vi "Hermite Interpolation 1D.vi"(9 "xi":dbl[](array[numeric]) format="%_6g", 10 "X":dbl[](array[numeric]), 11 "Y":dbl[](array[numeric])) -> (0 "error":i32, 1 "piecewise polynomial":T1 {"x locations" format="%.4g"; "coefficients" format="%.4g"}, 3 "yi":dbl[](array[numeric]) format="%_6g")   [LabVIEW 2010, in "NI_Gmath.lvlib"]
doc: "Performs one-dimensional interpolation using the cubic Hermite interpolation method based on the lookup table defined by <B>X</B> and <B>Y</B>."
uses:
  NI_Gmath.lvlib
  in_piecewise interp poly control.ctl
panel:
  # "Hermite Interpolation 1D"
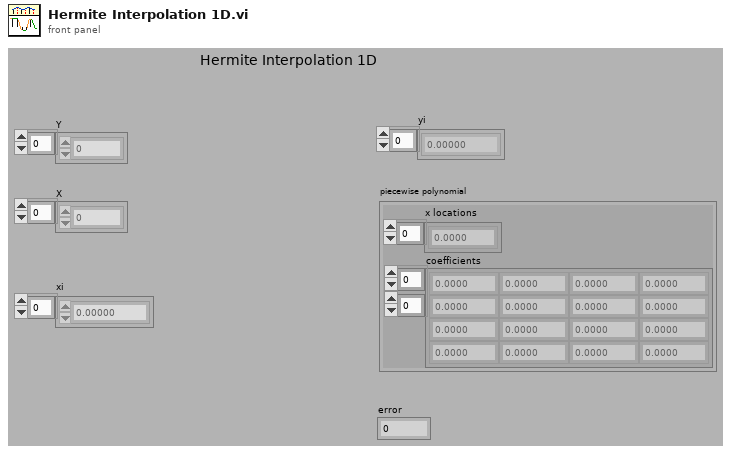
[diagram p1: front panel]
types:
  T1 = typedef "NI_Gmath.lvlib/in_piecewise interp poly control.ctl" = cluster{"x locations":dbl[], "coefficients":dbl[][]}
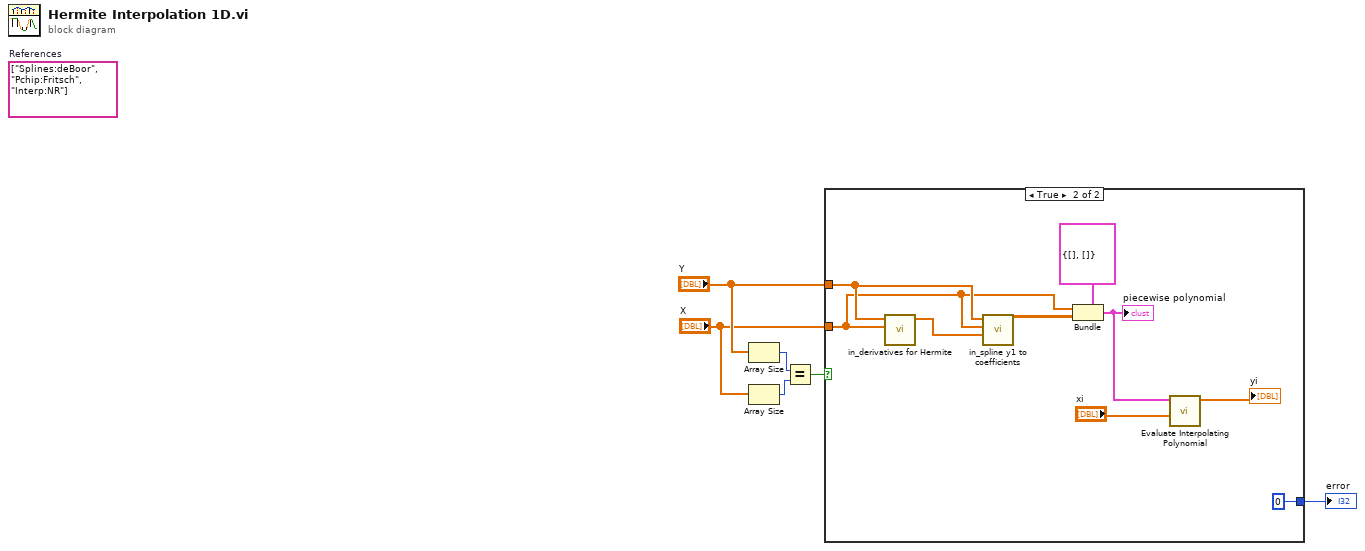
[diagram p0: block diagram]
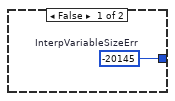
[diagram p2: hidden frame]
diagram:
  (unwired) string[] ["Splines:deBoor", "Pchip:Fritsch", "Interp:NR"]  # References
  n1 = Array Size(array="Y") -> (size(s)=w6:i32)
  n2 = Array Size(array="X") -> (size(s)=w5:i32)
  n3 = Equal?(x=w6, y=w5) -> (x = y?=w2:bool)
  n4 = case shown="True" w2 {
    tunnel: "Y" -> [_ w10]
    tunnel: "X" -> [_ w9]
    tunnel: [w7 0 ("error")] -> w1
    frame False {
      w7 = -20145  # InterpVariableSizeErr
    }
    frame True {
      n5 = call "in_derivatives for Hermite.vi"("Y[0..N]"=w10, "X[0..N]"=w9) -> ("Y deriv[0..N]"=w13:dbl[])  [unwired: 8 in]
      n6 = call "in_spline y1 to coefficients.vi"("Y1"=w13, "X"=w9, "Y"=w10) -> ("coefficients"=w16:dbl[][])  [unwired: 8 in]
      n7 = Bundle(cluster=T1 {"x locations"=[], "coefficients"=[]} ("interpolating polynomial"), "x locations"=w9, "coefficients"=w16) -> (w12:T1)
      "piecewise polynomial" <- w12
      n8 = call "Evaluate Interpolating Polynomial.vi"("xi"="xi", "piecewise polynomial"=w12) -> ("yi"=→"yi":dbl[])  [unwired: 8 in, 1 out]
    }
  }
  "error" <- w1
